vi "teleop.vi"(9 "Control Type":enum32{"Logitech Joysticks", "Logitech Gamepad"}(ring), 10 "Match Info":T1={"Autonomous Elapsed Seconds"=0.0, "TeleOp Elapsed Seconds"=0.0, "Disabled Elapsed Seconds"=0.0, "Visited Autonomous"=FALSE, "Visited TeleOp"=FALSE, "Visited Disabled"=FALSE, "Autonomous Settings"={"Autonomous Style"=enum."Independent", "VI Refnum"=refnum}}, 11 "Call Context":T2) -> ()   [LabVIEW 2011]
doc: "This VI is called for each TeleOp packet received from the DS where the robot is not disabled. It is often used to read from the joysticks and update I/O or to update setpoints for timed control loops. It should complete and return within 20 milliseconds or it may miss DS packets."
uses:
  <vilib>/Rock Robotics/WPI/DriverStation/WPI_DriverStationDerivedRobotMode.ctl
  <vilib>/Rock Robotics/WPI/DriverStation/WPI_DriverStationMatch Info.ctl
  <vilib>/Rock Robotics/WPI/Relay/WPI_RelayValue.ctl
  Robot Global Data.vi
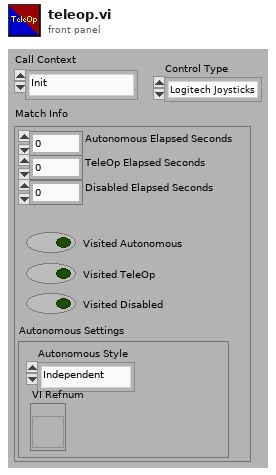
[diagram p1: front panel]
types:
  T1 = typedef "WPI_DriverStationMatch Info.ctl" = cluster{"Autonomous Elapsed Seconds":dbl, "TeleOp Elapsed Seconds":dbl, "Disabled Elapsed Seconds":dbl, "Visited Autonomous":bool, "Visited TeleOp":bool, "Visited Disabled":bool, "Autonomous Settings":cluster{"Autonomous Style":enum16{"Iterative", "Independent"}, "VI Refnum":refnum<vi>}}
  T2 = typedef "WPI_DriverStationDerivedRobotMode.ctl" = enum16{"Init", "Execute", "Stop"}
  T3 = typedef "WPI_JoystickDevRef.ctl" = cluster{"Device":T4}
  T4 = typedef "WPI_JoystickDeviceEnum.ctl" = enum16{"USB 1", "USB 2", "USB 3", "USB 4", "Kinect 1", "Kinect 2"}
  T5 = typedef "WPI_JoystickButtonState.ctl" = cluster{"Button 1":bool, "Button 2":bool, "Button 3":bool, "Button 4":bool, "Button 5":bool, "Button 6":bool, "Button 7":bool, "Button 8":bool, "Button 9":bool, "Button 10":bool, "Button 11":bool, "Button 12":bool}
  T6 = cluster{"axis 1 (x)":dbl, "axis 2 (y)":dbl, "axis 3 (throttle)":dbl, "axis 4":dbl, "axis 5":dbl, "axis 6":dbl}
  T7 = cluster{"Position":cluster{"X":dbl, "Y":dbl}, "Distance (ft)":dbl}[]
  T8 = typedef "WPI_MotorControlDeviceRef.ctl" = cluster{"DeviceStatus":errorcluster, "Type":enum16{"PWM", "CAN"}, "PWM":cluster{"Digital Module":T9, "PWM Channel":T10, "DeadBand":T11}, "CAN":cluster{"Device Number":u8, "Control Mode":T12, "Semaphore":T13, "Max Vout":dbl}, "Invert":bool, "TransformRef":T14, "InvTransformRef":T14}
  T9 = typedef "FPGA_TypedefDigitalModule.ctl" = enum16{"Digital Module 1", "Digital Module 2"}
  T10 = typedef "FPGA_DIOPWMChannel.ctl" = enum8{"PWM 1", "PWM 2", "PWM 3", "PWM 4", "PWM 5", "PWM 6", "PWM 7", "PWM 8", "PWM 9", "PWM 10", "Invalid"}
  T11 = typedef "WPI_PWMDeadband.ctl" = cluster{"Name":string, "maxPositivePwm":i32, "minPositivePwm":i32, "centerPwm":i32, "maxNegativePwm":i32, "minNegativePwm":i32, "angularRange":u16}
  T12 = typedef "WPI_CANJaguar_ControlMode.ctl" = enum8{"Percent VBus", "Current", "Speed", "Position", "Voltage"}
  T13 = typedef "Semaphore RefNum" = refnum<k1>
  T14 = typedef "WPI_PWMTransform_ConPane.ctl" = refnum<vi>
  T15 = typedef "WPI_RobotDriveDevRef.ctl" = cluster{"DevStatus":errorcluster, "Motors[]":T8[], "Square Inputs":bool, "Max Output":dbl, "Isochronous":bool}
  T16 = typedef "WPI_RelayValue.ctl" = enum16{"Off", "On", "Forward", "Reverse"}
  T17 = typedef "WPI_RelayDevRef.ctl" = cluster{"DevStatus":errorcluster, "Relay Channel":T18, "Digital Module":T9, "Relay Direction":T19}
  T18 = typedef "FPGA_DIORelayChannel.ctl" = enum8{"Relay 1", "Relay 2", "Relay 3", "Relay 4", "Relay 5", "Relay 6", "Relay 7", "Relay 8", "Invalid"}
  T19 = typedef "WPI_RelayDirection.ctl" = enum16{"Both directions", "Forward only", "Reverse only"}
  T20 = cluster{"Target Info[0]":cluster{"Position":cluster{"X":dbl, "Y":dbl}, "Distance (ft)":dbl}, "Target Info[1]":cluster{"Position":cluster{"X":dbl, "Y":dbl}, "Distance (ft)":dbl}, "Target Info[2]":cluster{"Position":cluster{"X":dbl, "Y":dbl}, "Distance (ft)":dbl}, "Target Info[3]":cluster{"Position":cluster{"X":dbl, "Y":dbl}, "Distance (ft)":dbl}, "Target Info[4]":cluster{"Position":cluster{"X":dbl, "Y":dbl}, "Distance (ft)":dbl}, "Target Info[5]":cluster{"Position":cluster{"X":dbl, "Y":dbl}, "Distance (ft)":dbl}, "Target Info[6]":cluster{"Position":cluster{"X":dbl, "Y":dbl}, "Distance (ft)":dbl}, "Target Info[7]":cluster{"Position":cluster{"X":dbl, "Y":dbl}, "Distance (ft)":dbl}, "Target Info[8]":cluster{"Position":cluster{"X":dbl, "Y":dbl}, "Distance (ft)":dbl}}
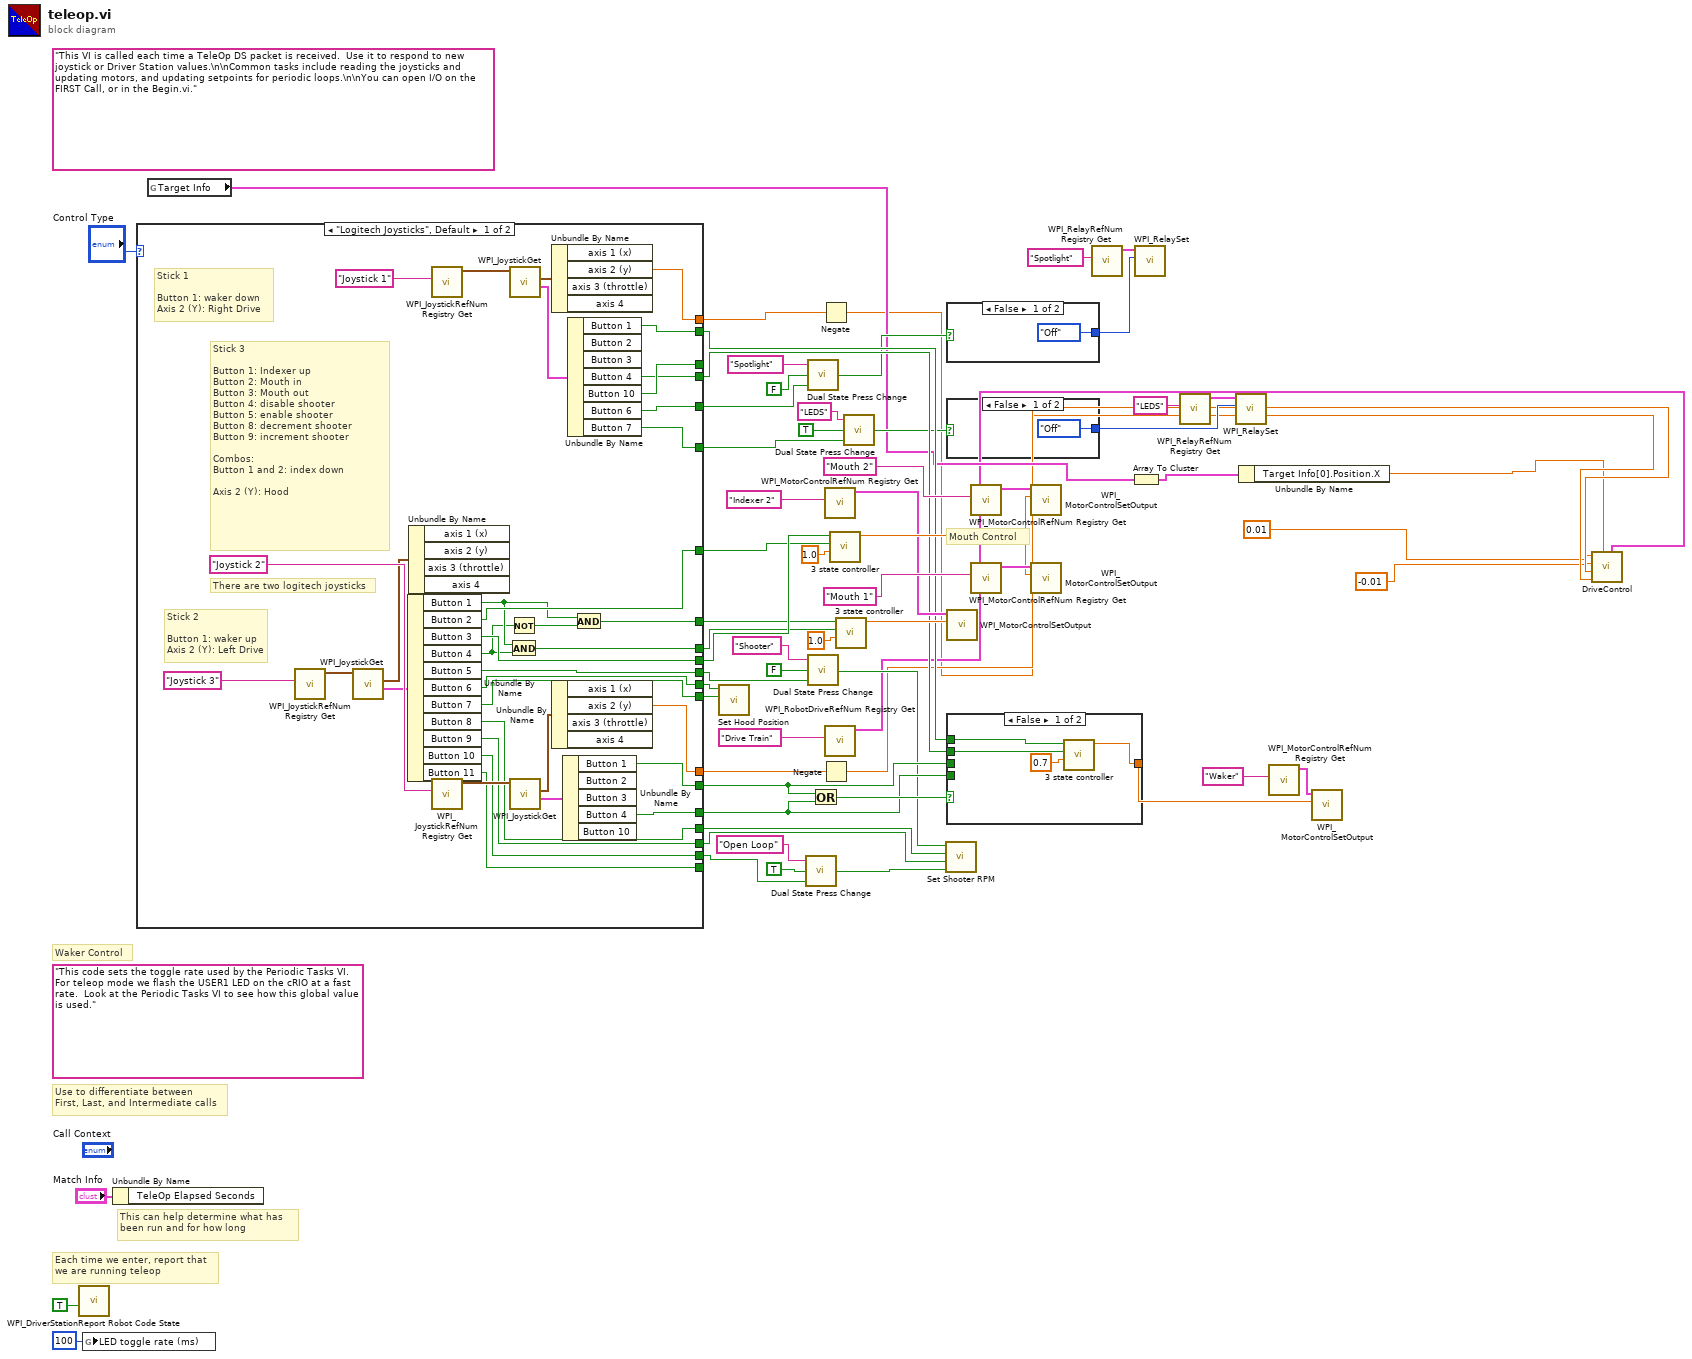
[diagram p0: block diagram]
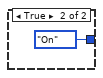
[diagram p2: hidden frame]
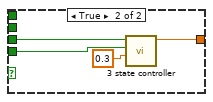
[diagram p3: hidden frame]
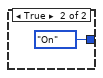
[diagram p4: hidden frame]
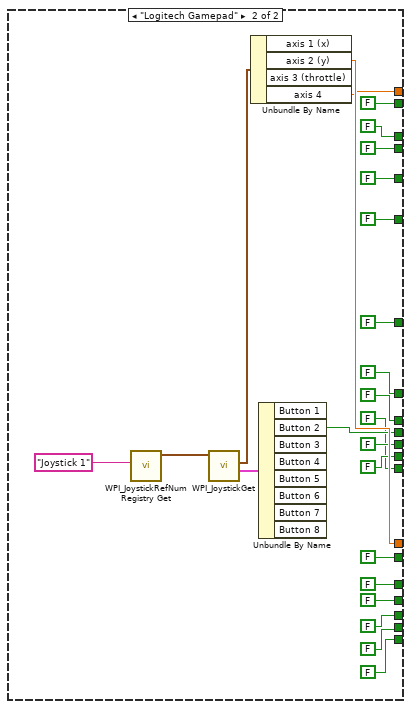
[diagram p5: hidden frame]
diagram:
  (unwired) "This code sets the toggle rate used by the Periodic Tasks VI.  For teleop mode we flash the USER1 LED on the cRIO at a fast rate.  Look at the Periodic Tasks VI to see how this global value is used."
  (unwired) "This VI is called each time a TeleOp DS packet is received.  Use it to respond to new joystick or Driver Station values.\n\nCommon tasks include reading the joysticks and updating motors, and updating setpoints for periodic loops.\n\nYou can open I/O on the FIRST Call, or in the Begin.vi."
  # "Waker Control"
  # "Mouth Control"
  # "Each time we enter, report that\nwe are running teleop"
  # "Use to differentiate between\nFirst, Last, and Intermediate calls"
  # "This can help determine what has\nbeen run and for how long"
  n1 = call <vilib>:"WPI_DriverStationReport Robot Code State.vi"("TeleOp"=TRUE ("Autonomous")) -> ()  [unwired: 10 in, 1 out]
  n2 = global write "Robot Global Data.vi" "LED toggle rate (ms)"(u32 100 ("LED ms toggle rate")) -> ()
  n3 = Unbundle By Name("Match Info") -> ()  [unwired: 1 out]
  n4 = case shown="\"Logitech Joysticks\", Default" "Control Type" {
    tunnel: [w90 w122] -> w43
    tunnel: [w89 w121] -> w42
    tunnel: [w83 w120] -> w57
    tunnel: [w84 FALSE ("Button 5")] -> w29
    tunnel: [w81 FALSE ("Button 3")] -> w53
    tunnel: [w82 FALSE ("Button 11")] -> _
    tunnel: [w80 FALSE ("Button 6")] -> w20
    tunnel: [w79 FALSE ("Button 5")] -> w15
    tunnel: [w78 FALSE ("Button 8")] -> w49
    tunnel: [w77 FALSE ("Button 9")] -> w48
    tunnel: [w76 FALSE] -> w47
    tunnel: [w72 FALSE] -> w46
    tunnel: [w71 FALSE ("Button 6")] -> w45
    tunnel: [w70 FALSE ("Button 7")] -> w44
    tunnel: [w69 FALSE ("Button 10")] -> w9
    tunnel: [w68 FALSE ("Button 1")] -> w33
    tunnel: [w67 FALSE ("Button 4")] -> w32
    tunnel: [w66 FALSE ("Button 10")] -> _
    tunnel: [w65 FALSE ("Button 4")] -> w30
    tunnel: [w64 FALSE ("Button 7")] -> w23
    frame "Logitech Joysticks", Default {
      # "Stick 3\n\nButton 1: Indexer up\nButton 2: Mouth in\nButton 3: Mouth out\nButton 4: disable shooter\nButton 5: enable shooter\nButton 8: decrement shooter\nButton 9: increment shooter\n\nCombos:\nButton 1 and 2: index down\n \nAxis 2 (Y): Hood"
      # "Stick 2\n\nButton 1: waker up\nAxis 2 (Y): Left Drive"
      # "Stick 1\n\nButton 1: waker down\nAxis 2 (Y): Right Drive"
      # "There are two logitech joysticks"
      n5 = call <vilib>:"WPI_JoystickRefNum Registry Get.vi"("refnum name"="Joystick 3") -> ("JoystickDevRef"=w87:T3)  [unwired: 9 in, 1 out]
      n6 = call <vilib>:"WPI_JoystickGet.vi"("JoystickDevRef"=w87) -> ("Buttons"=w85:T5, "Axes"=w86:T6)  [unwired: 4 in, 1 out]
      n7 = Unbundle By Name(w85) -> ("Button 1"=w74:bool, "Button 2"=w81:bool, "Button 3"=w83:bool, "Button 4"=w73:bool, "Button 5"=w79:bool, "Button 6"=w71:bool, "Button 7"=w70:bool, "Button 8"=w78:bool, "Button 9"=w77:bool, "Button 10"=w69:bool, "Button 11"=w82:bool)
      n8 = Unbundle By Name(w86) -> ()  [unwired: 4 out]
      n9 = call <vilib>:"WPI_JoystickRefNum Registry Get.vi"("refnum name"="Joystick 1") -> ("JoystickDevRef"=w96:T3)  [unwired: 9 in, 1 out]
      n10 = call <vilib>:"WPI_JoystickRefNum Registry Get.vi"("refnum name"="Joystick 2") -> ("JoystickDevRef"=w97:T3)  [unwired: 9 in, 1 out]
      n11 = Not(x=w73) -> (.not. x?=w75:bool)
      n12 = And(x=w74, y=w73) -> (x .and. y?=w72:bool)
      n13 = call <vilib>:"WPI_JoystickGet.vi"("JoystickDevRef"=w96) -> ("Buttons"=w92:T5, "Axes"=w91:T6)  [unwired: 4 in, 1 out]
      n14 = call <vilib>:"WPI_JoystickGet.vi"("JoystickDevRef"=w97) -> ("Buttons"=w94:T5, "Axes"=w93:T6)  [unwired: 4 in, 1 out]
      n15 = Unbundle By Name(w91) -> ("axis 2 (y)"=w89:dbl)  [unwired: 3 out]
      n16 = Unbundle By Name(w93) -> ("axis 2 (y)"=w90:dbl)  [unwired: 3 out]
      n17 = Unbundle By Name(w94) -> ("Button 1"=w68:bool, "Button 4"=w67:bool)  [unwired: 3 out]
      n18 = Unbundle By Name(w92) -> ("Button 1"=w84:bool, "Button 4"=w65:bool, "Button 10"=w66:bool, "Button 6"=w80:bool, "Button 7"=w64:bool)  [unwired: 2 out]
      n19 = And(x=w74, y=w75) -> (x .and. y?=w76:bool)
    }
    frame "Logitech Gamepad" {
      n20 = call <vilib>:"WPI_JoystickRefNum Registry Get.vi"("refnum name"="Joystick 1") -> ("JoystickDevRef"=w118:T3)  [unwired: 9 in, 1 out]
      n21 = call <vilib>:"WPI_JoystickGet.vi"("JoystickDevRef"=w118) -> ("Buttons"=w116:T5, "Axes"=w117:T6)  [unwired: 4 in, 1 out]
      n22 = Unbundle By Name(w117) -> ("axis 2 (y)"=w122:dbl, "axis 4"=w121:dbl)  [unwired: 2 out]
      n23 = Unbundle By Name(w116) -> ("Button 2"=w120:bool)  [unwired: 7 out]
    }
  }
  n24 = global read "Robot Global Data.vi" "Target Info"() -> (w8:T7)
  n25 = call "Set Hood Position.vi"("Increment"=w44, "Decrement"=w45) -> ()  [unwired: 10 in]
  n26 = call "Dual State Press Change.vi"("Enable/Disable"=w9, "Initial"=TRUE, "Value Name"="Open Loop") -> ("Enabled"=w10:bool)
  n27 = call "Dual State Press Change.vi"("Enable/Disable"=w20, "Initial"=FALSE, "Value Name"="Spotlight") -> ("Enabled"=w17:bool)
  n28 = call "Dual State Press Change.vi"("Enable/Disable"=w15, "Initial"=FALSE, "Value Name"="Shooter") -> ("Enabled"=w13:bool)
  n29 = Or(x=w33, y=w32) -> (x .or. y?=w34:bool)
  n30 = Negate(x=w42) -> (-x=w4:dbl)
  n31 = Negate(x=w43) -> (-x=w5:dbl)
  n32 = call <vilib>:"WPI_MotorControlRefNum Registry Get.vi"("refnum name"="Indexer 2") -> ("MotorControlDevRef"=w38:T8)  [unwired: 9 in, 1 out]
  n33 = call <vilib>:"WPI_RobotDriveRefNum Registry Get.vi"("refnum name"="Drive Train") -> ("RobotDriveDevRef"=w6:T15)  [unwired: 9 in, 1 out]
  n34 = call "3 state controller.vi"("Power"=1.0, "Backward"=w53, "Forward"=w57) -> ("Numeric"=w54:dbl)  [unwired: 8 in]
  n35 = call "3 state controller.vi"("Power"=1.0, "Backward"=w46, "Forward"=w47) -> ("Numeric"=w37:dbl)  [unwired: 8 in]
  n36 = call "Dual State Press Change.vi"("Enable/Disable"=w23, "Initial"=TRUE, "Value Name"="LEDS") -> ("Enabled"=w18:bool)
  n37 = call "Set Shooter RPM.vi"("Open Loop"=w10, "Increment"=w48, "Decrement"=w49, "Shooter Enabled"=w13) -> ()  [unwired: 8 in]
  n38 = case shown="False" w17 {
    tunnel: [WPI_RelayValue."Off" ("RelayValue") WPI_RelayValue."On" ("RelayValue")] -> w35
    frame False {
    }
    frame True {
    }
  }
  n39 = case shown="False" w18 {
    tunnel: [WPI_RelayValue."Off" ("RelayValue") WPI_RelayValue."On" ("RelayValue")] -> w25
    frame False {
    }
    frame True {
    }
  }
  n40 = call <vilib>:"WPI_MotorControlSetOutput.vi"("Output"=w37, "MotorControlDevRef"=w38) -> ()  [unwired: 8 in, 2 out]
  n41 = case shown="False" w34 {
    tunnel: w33 -> [_ w134]
    tunnel: w32 -> [_ w133]
    tunnel: [w127 w131] -> w28
    tunnel: w30 -> [w129 _]
    tunnel: w29 -> [w130 _]
    frame False {
      n42 = call "3 state controller.vi"("Power"=0.7, "Backward"=w129, "Forward"=w130) -> ("Numeric"=w127:dbl)  [unwired: 8 in]
    }
    frame True {
      n43 = call "3 state controller.vi"("Power"=0.3, "Backward"=w133, "Forward"=w134) -> ("Numeric"=w131:dbl)  [unwired: 8 in]
    }
  }
  n44 = call <vilib>:"WPI_MotorControlRefNum Registry Get.vi"("refnum name"="Mouth 2") -> ("MotorControlDevRef"=w55:T8)  [unwired: 9 in, 1 out]
  n45 = call <vilib>:"WPI_MotorControlRefNum Registry Get.vi"("refnum name"="Mouth 1") -> ("MotorControlDevRef"=w58:T8)  [unwired: 9 in, 1 out]
  n46 = call <vilib>:"WPI_MotorControlSetOutput.vi"("Output"=w54, "MotorControlDevRef"=w55) -> ()  [unwired: 8 in, 2 out]
  n47 = call <vilib>:"WPI_MotorControlSetOutput.vi"("Output"=w54, "MotorControlDevRef"=w58) -> ()  [unwired: 8 in, 2 out]
  n48 = call <vilib>:"WPI_RelayRefNum Registry Get.vi"("refnum name"="Spotlight") -> ("RelayDevRef"=w50:T17)  [unwired: 9 in, 1 out]
  n49 = Array To Cluster(array=w8) -> (cluster=w7:T20)
  n50 = call <vilib>:"WPI_RelaySet.vi"("RelayValue"=w35, "RelayDevRef"=w50) -> ()  [unwired: 8 in, 2 out]
  n51 = call <vilib>:"WPI_RelayRefNum Registry Get.vi"("refnum name"="LEDS") -> ("RelayDevRef"=w27:T17)  [unwired: 9 in, 1 out]
  n52 = call <vilib>:"WPI_RelaySet.vi"("RelayValue"=w25, "RelayDevRef"=w27) -> ()  [unwired: 8 in, 2 out]
  n53 = Unbundle By Name(w7) -> ("Target Info[0].Position.X"=w1:dbl)
  n54 = call <vilib>:"WPI_MotorControlRefNum Registry Get.vi"("refnum name"="Waker") -> ("MotorControlDevRef"=w31:T8)  [unwired: 9 in, 1 out]
  n55 = call <vilib>:"WPI_MotorControlSetOutput.vi"("Output"=w28, "MotorControlDevRef"=w31) -> ()  [unwired: 8 in, 2 out]
  n56 = call "DriveControl.vi"("RobotDriveDevRef"=w6, "Xvalue of Target"=w1, "Right axis value"=w4, "Left axis value"=w5, "Lower Bound"=-0.01, "Upper Bound"=0.01) -> ()  [unwired: 6 in]
